vi "magnitude_mat.vi"(4 "vector":T1) -> (1 "vector magnitude":dbl)   [LabVIEW 2013]
uses:
  <vilib>/Analysis/Matrix/Datatypes/RealMatrix.ctl
  <vilib>/Analysis/Matrix/NI_Matrix.lvlib
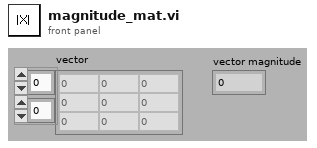
[diagram p1: front panel]
types:
  T1 = typedef "NI_Matrix.lvlib/RealMatrix.ctl" = dbl[][]
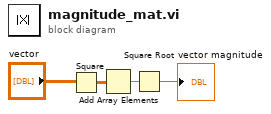
[diagram p0: block diagram]
diagram:
  n1 = Square(x="vector") -> (x^2=w4:T1)
  n2 = Add Array Elements(numeric array=w4) -> (sum=w3:dbl)
  n3 = Square Root(x=w3) -> (sqrt(x)=→"vector magnitude":dbl)
